vi "error log tester independent.vi"   [LabVIEW 2017]
uses:
  Global Variables/General Globals.vi
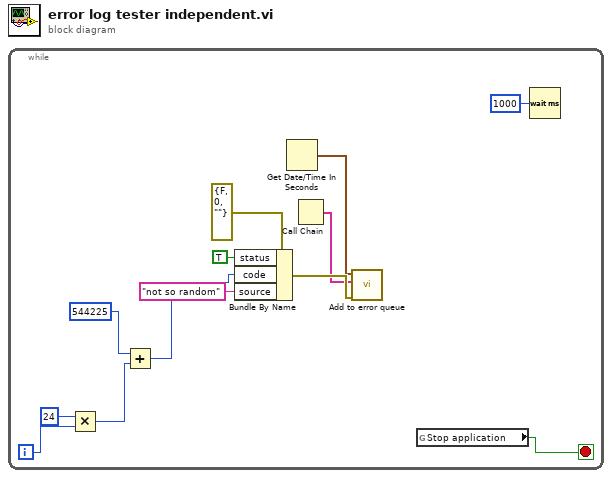
[diagram p0: block diagram]
diagram:
  n1 = while {
    i -> [w10]
    stop <- w1 stop-if-true
    n2 = Multiply(x=24, y=w10) -> (x*y=w7:i32)
    n3 = Add(x=544225, y=w7) -> (x+y=w6:i32)
    n4 = Bundle By Name(cluster=errorcluster {"status"=FALSE, "code"=0, "source"=""} ("error in (no error)"), "status"=TRUE, "code"=w6, "source"="not so random") -> (w4:errorcluster)
    n5 = Get Date/Time In Seconds() -> (seconds since 1Jan1904=w2:timestamp)
    n6 = Call Chain() -> (call chain=w3:string[])
    n7 = call "Add to error queue.vi"("error in (no error)"=w4, "Call Chain"=w3, "Time Stamp"=w2) -> ()  [unwired: 9 in]
    n8 = global read "General Globals.vi" "Stop application"() -> (w1:bool)
    n9 = Wait (ms)(milliseconds to wait=u32 1000) -> ()  [unwired: 1 out]
  }
